vi "CLD 10 Unbundle data SubVI.vi"(8 "Fehler (Eingang, kein Fehler)":errorcluster, 10 "Nr. des aktuellen Zustands":i32, 11 "[Daten, Eingang]":T1[](array[typedef])) -> (0 "Fehler (Ausgang)":errorcluster, 1 "Zustand 3":bool, 2 "Zustand 2":bool, 3 "[Daten, Ausgang]":T1[](array[typedef]), 4 "Nächste Verweildauer":dbl, 5 "Zustand 1":bool, 6 "Verweildauer":dbl)   [LabVIEW 2014]
doc: "CLD-Übung 10\n\nMit diesem Sub-VI wird das Auslesen von Daten aus dem Cluster-Array in der Hauptapplikation vereinfacht."
uses:
  CLD 10 CSV file data structure.ctl
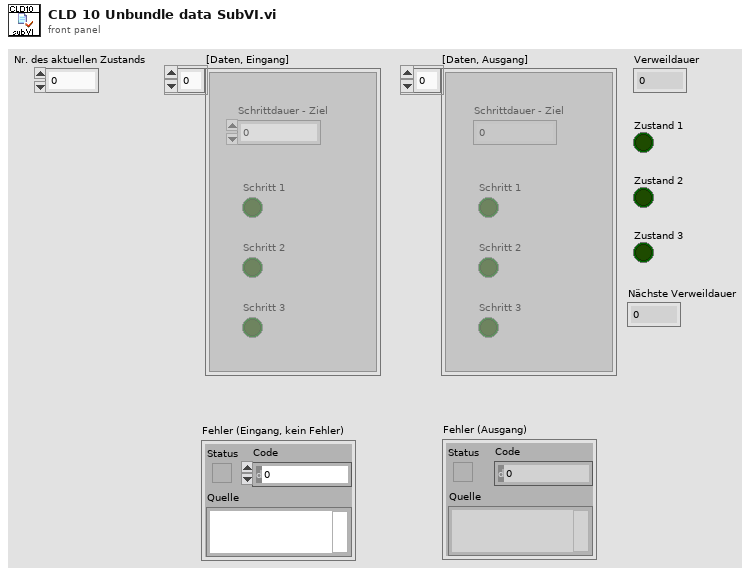
[diagram p1: front panel]
types:
  T1 = typedef "CLD 10 CSV file data structure.ctl" = cluster{"Schrittdauer - Ziel":i32, "Schritt 1":bool, "Schritt 2":bool, "Schritt 3":bool}
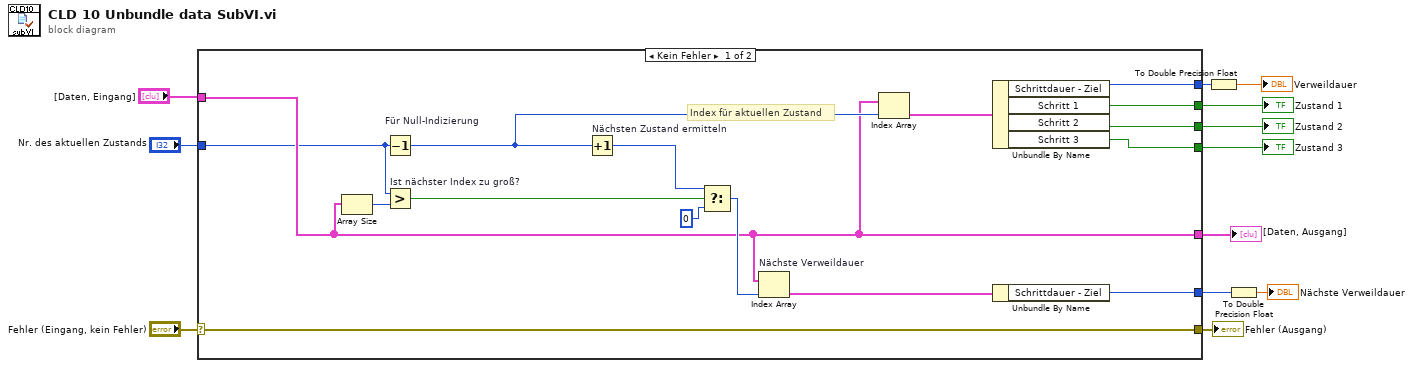
[diagram p0: block diagram]
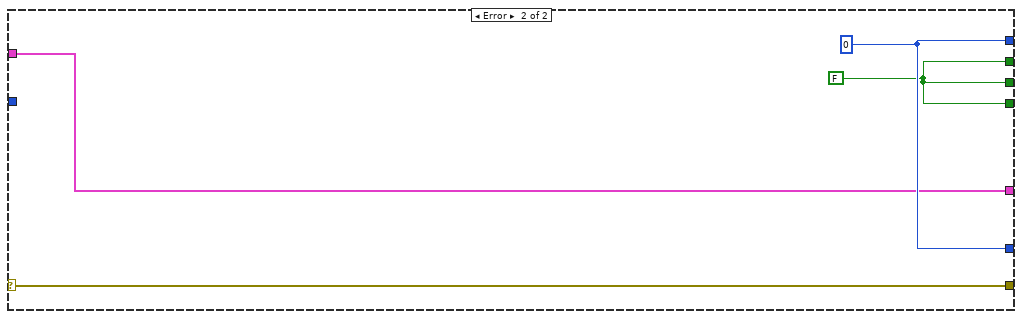
[diagram p2: hidden frame]
diagram:
  n1 = case shown="Kein Fehler" "Fehler (Eingang, kein Fehler)" {
    selector: "Fehler (Eingang, kein Fehler)" -> [w15 w32]
    tunnel: [w27 w30] -> w12
    tunnel: [w26 w30] -> w11
    tunnel: [w25 w30] -> w10
    tunnel: [w24 w31] -> w9
    tunnel: "[Daten, Eingang]" -> [w14 w29]
    tunnel: [w17 w31] -> w6
    tunnel: [w15 w32] -> w3
    tunnel: [w14 w29] -> w2
    tunnel: "Nr. des aktuellen Zustands" -> [w13 _]
    frame No Error {
      # "Index für aktuellen Zustand"
      n2 = Array Size(array=w14) -> (size(s)=w20:i32)
      n3 = Decrement "Für Null-Indizierung"(x=w13) -> (x-1=w16:i32)
      n4 = Greater? "Ist nächster Index zu groß?"(x=w13, y=w20) -> (0:w23:bool)
      n5 = Increment "Nächsten Zustand ermitteln"(x=w16) -> (x+1=w19:i32)
      n6 = Select(t=w19, s=w23, f=0) -> (s? t:f=w21:i32)
      n7 = Index Array "Nächste Verweildauer"(array=w14, index=w21) -> (element=w18:T1)
      n8 = Index Array(array=w14, index=w16) -> (element=w28:T1)
      n9 = Unbundle By Name(w28) -> ("Schrittdauer - Ziel"=w24:i32, "Schritt 1"=w27:bool, "Schritt 2"=w26:bool, "Schritt 3"=w25:bool)
      n10 = Unbundle By Name(w18) -> ("Schrittdauer - Ziel"=w17:i32)
    }
    frame Error {
      w30 = FALSE ("Zustand 1")
      w31 = 0 ("Verweildauer")
    }
  }
  "Zustand 1" <- w12
  "Zustand 2" <- w11
  "Zustand 3" <- w10
  "Fehler (Ausgang)" <- w3
  "[Daten, Ausgang]" <- w2
  n11 = To Double Precision Float(number=w9) -> (double precision float=→"Verweildauer":dbl)
  n12 = To Double Precision Float(number=w6) -> (double precision float=→"Nächste Verweildauer":dbl)
